vi "format_message.vi"(1 "messge":string) -> (0 "concatenated string":string)   [LabVIEW 2013, in "TCP_IP.lvclass"]
uses:
  TCP_IP.lvclass
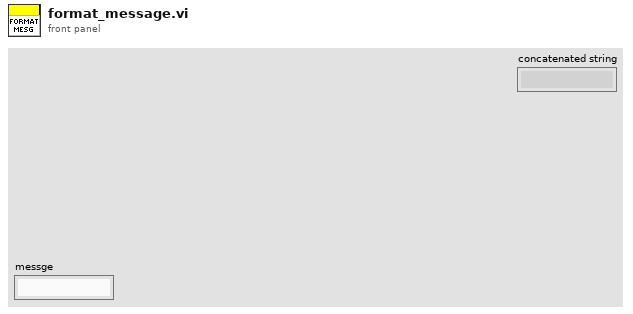
[diagram p1: front panel]
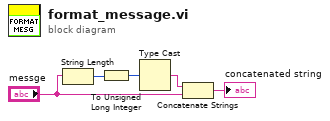
[diagram p0: block diagram]
diagram:
  n1 = String Length(string="messge") -> (length=w2:i32)
  n2 = To Unsigned Long Integer(number=w2) -> (unsigned 32bit integer=w5:u32)
  n3 = Type Cast(x=w5) -> (*(type *) &x=w4:string)  [unwired: 1 in]
  n4 = Concatenate Strings(w4, "messge") -> (→"concatenated string":string)
